vi "Calculate H Matrix.vi"(10 "Measured Points":dbl[][](array[numeric])) -> (0 "World corner points (out)":dbl[][](array[numeric])=[[-3.25, -3.25, 0.0], [3.25, -3.25, 0.0], [3.25, 3.25, 0.0], [-3.25, 3.25, 0.0]], 1 "Euclidean Error":dbl[](array[numeric]) format="%#_6f", 2 "Homography H":T1)   [LabVIEW 2025]
uses:
  <vilib>/Analysis/Matrix/Datatypes/RealMatrix.ctl
  <vilib>/Analysis/7linalg.llb/SVD Option.ctl
  <vilib>/Analysis/7linalg.llb/Real SVD Decomposition.vi
  <vilib>/Analysis/Matrix/Numeric/Conversions/Matrix To Array - RM.vi
  <vilib>/Analysis/NI_AALPro.lvlib
  <vilib>/Analysis/Matrix/NI_Matrix.lvlib
panel:
  out "Projected Points":dbl[][](array[numeric])
  out "Matrix V":T1
  out "Exact numeric A Matrix":dbl[][](array[numeric])
  in  "World corner points":dbl[][](array[numeric])=[[-3.25, -3.25, 0.0], [3.25, -3.25, 0.0], [3.25, 3.25, 0.0], [-3.25, 3.25, 0.0]]
  # "Bottom Left"
  # "Bottom Right"
  # "Top Right"
  # "Top Left"
  # "Bottom Left"
  # "Bottom Right"
  # "Top Right"
  # "Top Left"
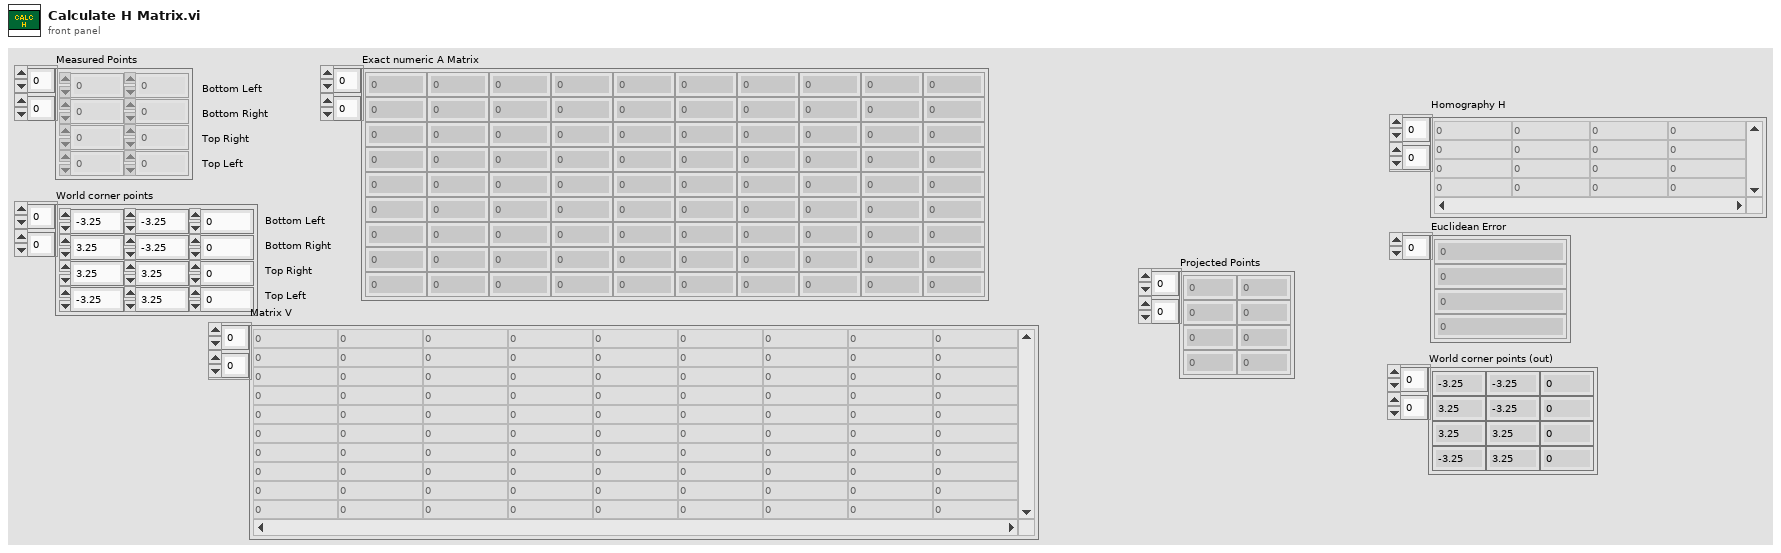
[diagram p1: front panel]
types:
  T1 = typedef "NI_Matrix.lvlib/RealMatrix.ctl" = dbl[][]
  T2 = typedef "NI_AALPro.lvlib/SVD Option.ctl" = u16
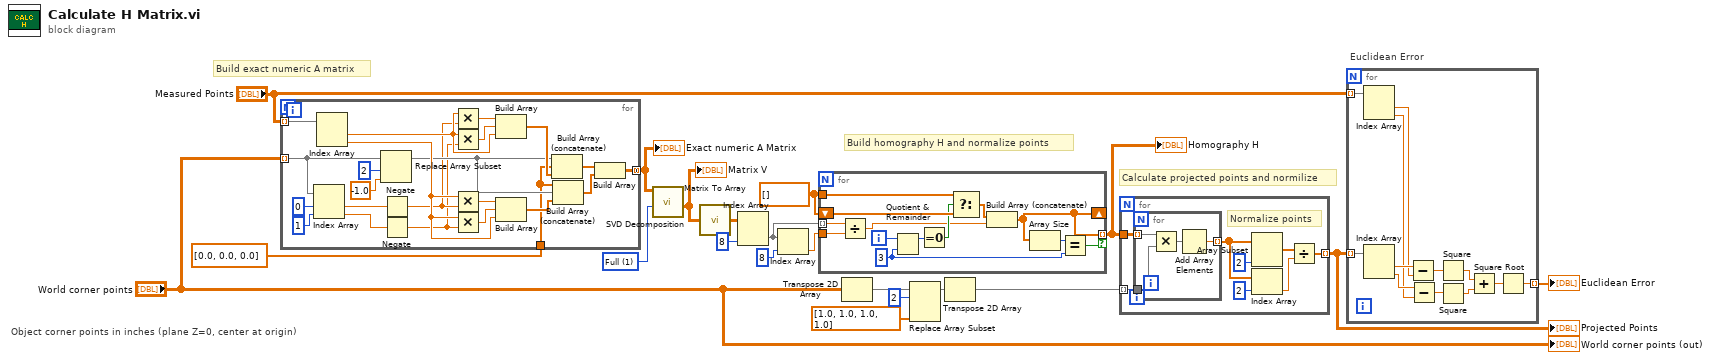
[diagram p0: block diagram]
diagram:
  w16 = T2 1 items=["Thin", "Full"] ("SVD option")
  w18 = dbl[] []
  # "Object corner points in inches (plane Z=0, center at origin)"
  # "Calculate projected points and normilize"
  # "Build exact numeric A matrix"
  # "Euclidean Error"
  # "Build homography H and normalize points"
  n1 = for {
    tunnel: "Measured Points" -> [w43] mode=indexing
    tunnel: "World corner points" -> [w31] mode=indexing
    tunnel: [w40] -> w19 mode=concatenating
    tunnel: dbl[] [0.0, 0.0, 0.0] -> [w23]
    n2 = Index Array(array=w31, index #1=0 ("index"), index #2=1 ("index")) -> (element #1=w37:dbl, element #2=w36:dbl)
    n3 = Index Array(array=w43) -> (element #1=w33:dbl, element #2=w27:dbl)  [unwired: 2 in]
    n4 = Replace Array Subset(array=w31, new element=-1.0 ("new element/subarray"), index=2) -> (w24:dbl[])
    n5 = Negate(x=w37) -> (-x=w22:dbl)
    n6 = Negate(x=w36) -> (-x=w21:dbl)
    n7 = Multiply(x=w33, y=w22) -> (x*y=w35:dbl)
    n8 = Multiply(x=w33, y=w21) -> (x*y=w34:dbl)
    n9 = Multiply(x=w27, y=w22) -> (x*y=w38:dbl)
    n10 = Multiply(x=w27, y=w21) -> (x*y=w39:dbl)
    n11 = Build Array(w35, w34, w33) -> (w32:dbl[])
    n12 = Build Array(w38, w39, w27) -> (w30:dbl[])
    n13 = Build Array (concatenate)(w24, w23, w32) -> (w42:dbl[])
    n14 = Build Array (concatenate)(w23, w24, w30) -> (w41:dbl[])
    n15 = Build Array(w42, w41) -> (w40:dbl[][])
  }
  "Exact numeric A Matrix" <- w19
  n16 = call-poly <vilib>:"SVD Decomposition.vi"("SVD option"=w16, "A"=w19) -> ("Matrix V"=w15:T1)  [unwired: 5 in, 4 out]
  "Matrix V" <- w15
  n17 = call-poly <vilib>:"Matrix To Array.vi"("Real Matrix"=w15) -> ("Real 2D Array"=w14:dbl[][])
  n18 = Index Array(array=w14, index (col)=8) -> (element=w12:dbl[])  [unwired: 1 in]
  n19 = Index Array(array=w12, index=8) -> (element=w13:dbl)
  n20 = for {
    tunnel: w12 -> [w56] mode=indexing
    shift-right: [w49] -> _
    shift-left: w18 -> [w54]
    tunnel: [w49] -> w10 mode=indexing if=w46
    tunnel: w18 -> [w55]
    tunnel: w13 -> [w44]
    i -> [w52]
    w47 = 3 ("y")
    n21 = Divide(x=w56, y=w44) -> (x/y=w45:dbl)
    n22 = Quotient & Remainder(x=w52, y=w47) -> (x-y*floor(x/y)=w51:i32)  [unwired: 1 out]
    n23 = Equal To 0?(x=w51) -> (x = 0?=w50:bool)
    n24 = Select(t=w55, s=w50, f=w54) -> (s? t:f=w53:dbl[])
    n25 = Build Array (concatenate)(w53, w45) -> (w49:dbl[])
    n26 = Array Size(array=w49) -> (size(s)=w48:i32)
    n27 = Equal?(x=w48, y=w47) -> (x = y?=w46:bool)
  }
  "Homography H" <- w10
  n28 = Transpose 2D Array(2D array="World corner points") -> (transposed array=w7:dbl[][])
  n29 = Replace Array Subset(array=w7, new element=dbl[] [1.0, 1.0, 1.0, 1.0] ("new element/subarray"), index (row)=2) -> (w9:dbl[][])  [unwired: 1 in]
  n30 = Transpose 2D Array(2D array=w9) -> (transposed array=w4:dbl[][])
  n31 = for {
    tunnel: w10 -> [w64]
    tunnel: w4 -> [w63] mode=indexing
    tunnel: [w57] -> w5 mode=indexing
    # "Normalize points"
    n32 = for {
      tunnel: w64 -> [w67] mode=indexing
      tunnel: w63 -> [w68]
      tunnel: [w65] -> w61 mode=indexing
      n33 = Multiply(x=w67, y=w68) -> (x*y=w66:dbl[])
      n34 = Add Array Elements(numeric array=w66) -> (sum=w65:dbl)
    }
    n35 = Array Subset(array=w61, length=2) -> (w59:dbl[])  [unwired: 1 in]
    n36 = Index Array(array=w61, index=2) -> (element=w58:dbl)
    n37 = Divide(x=w59, y=w58) -> (x/y=w57:dbl[])
  }
  "Projected Points" <- w5
  n38 = for {
    tunnel: w5 -> [w79] mode=indexing
    tunnel: "Measured Points" -> [w80] mode=indexing
    tunnel: [w69] -> w2 mode=indexing
    n39 = Index Array(array=w80) -> (element #1=w77:dbl, element #2=w74:dbl)  [unwired: 2 in]
    n40 = Index Array(array=w79) -> (element #1=w78:dbl, element #2=w75:dbl)  [unwired: 2 in]
    n41 = Subtract(x=w78, y=w77) -> (x-y=w76:dbl)
    n42 = Subtract(x=w75, y=w74) -> (x-y=w73:dbl)
    n43 = Square(x=w76) -> (x^2=w71:dbl)
    n44 = Square(x=w73) -> (x^2=w72:dbl)
    n45 = Add(x=w71, y=w72) -> (x+y=w70:dbl)
    n46 = Square Root(x=w70) -> (sqrt(x)=w69:dbl)
  }
  "Euclidean Error" <- w2
  "World corner points (out)" <- "World corner points"
